vi "Create VariantMessage.vi"(8 "error in (no error)":errorcluster, 10 "Message Data":variant, 11 "Message Name":string) -> (0 "error out":errorcluster, 3 "VariantMessage Out":refnum<class "VariantMessage.lvclass">)   [LabVIEW 2009, in "LapDog.Messaging.v2.NativeTypes.lvlib" / "VariantMessage.lvclass"]
doc: "Returns a VariantMessage object with the given name.\n\nThis method executes regardless of the error in state."
uses:
  VariantMessage.lvclass
  VariantMessage.lvclass/VariantMessage.ctl
  Messaging.v2/MessageObject/Message.lvclass
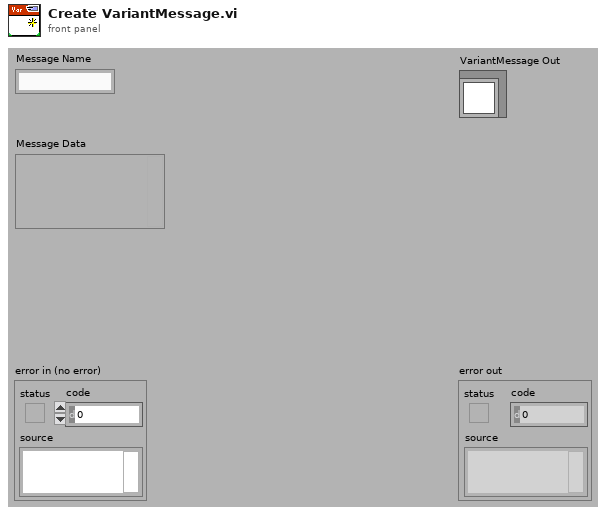
[diagram p1: front panel]
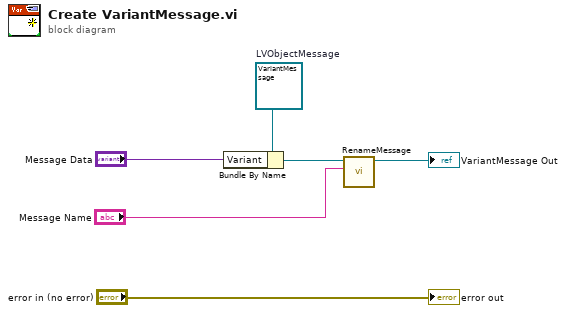
[diagram p0: block diagram]
diagram:
  w1 = refnum<class "VariantMessage.lvclass"> refnum  # LVObjectMessage
  n1 = Bundle By Name(cluster=w1, "Variant"="Message Data") -> (w4:refnum<class "VariantMessage.lvclass">)
  n2 = call "RenameMessage.vi"("Message Name"="Message Name", "Message in"=w4) -> ("Message out"=→"VariantMessage Out":refnum<class "VariantMessage.lvclass">)  [unwired: 8 in, 1 out]
  "error out" <- "error in (no error)"
